vi "GFITS_NetServer2.vi"(7 "ID":string, 8 "error in (no error)":errorcluster, 9 "notifier In":refnum<notifier>, 10 "messages from sock":refnum<queue>, 11 "listener ID":refnum<k5>) -> (0 "error out":errorcluster)   [LabVIEW 2016]
uses:
  DHS_TCPSERVER_MsgStruct.ctl
panel:
  in  "ResponseStruct":T1
  out "sock ID":refnum<k5>
  out "stop":bool
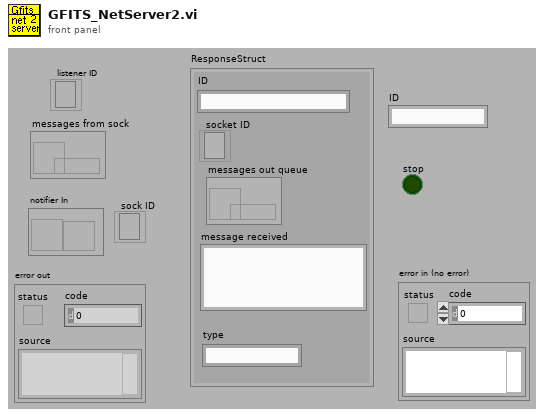
[diagram p1: front panel]
types:
  T1 = typedef "DHS_TCPSERVER_MsgStruct.ctl" = cluster{"ID":string, "socket ID":refnum<k5>, "messages out queue":refnum<queue>, "message received":string, "type":string}
  T2 = enum16{"Standard", "Buffered", "CRLF", "Immediate"}
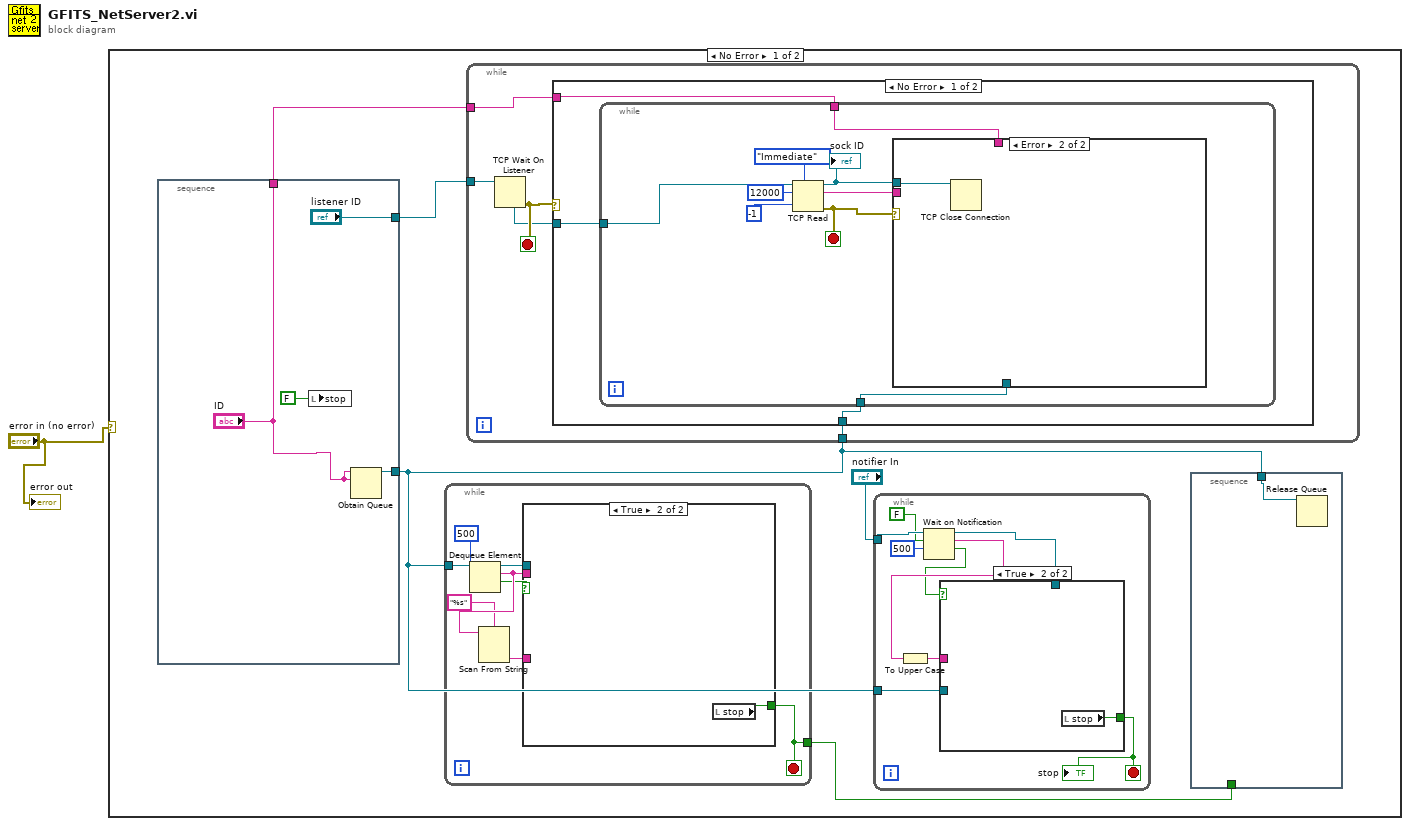
[diagram p0: block diagram]
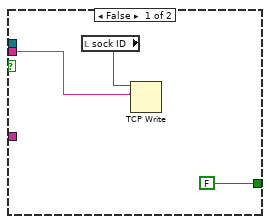
[diagram p2: hidden frame]
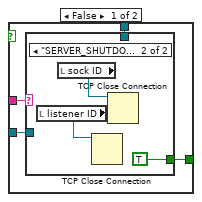
[diagram p3: hidden frame]
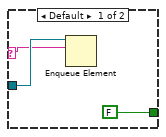
[diagram p4: hidden frame]
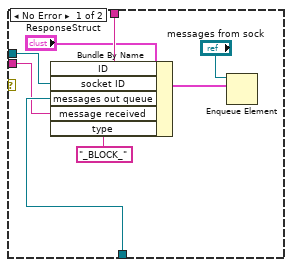
[diagram p5: hidden frame]
diagram:
  n1 = case shown="No Error" "error in (no error)" {
    frame No Error {
      n2 = stacked-sequence {
        tunnel: [w11] -> w2
        tunnel: ["listener ID"] -> w5
        tunnel: ["ID"] -> w4
        frame #0 {
          n3 = local write "stop"(FALSE ("stop")) -> ()
          n4 = Obtain Queue(name (unnamed)="ID", element data type="ID") -> (queue out=w11:refnum<queue>)  [unwired: 3 in, 2 out]
        }
      }
      n5 = while {
        tunnel: w2 -> [w19]
        tunnel: [w12] -> w3
        stop <- w12 stop-if-true
        n6 = Dequeue Element(queue=w19, timeout in ms (-1)=500) -> (queue out=w15:refnum<queue>, element=w18:string, timed out?=w14:bool)  [unwired: 1 in, 1 out]
        n7 = Scan From String(format string="%s", input string=w18) -> (output 1=w16:string)  [unwired: 2 in, 4 out]
        n8 = case shown="True" w14 {
          tunnel: w18 -> [w22 _]
          tunnel: w16 -> [_ _]
          tunnel: [FALSE w23] -> w12
          tunnel: w15 -> [_ _]
          frame False {
            n9 = local read "sock ID"() -> (w20:refnum<k5>)
            n10 = TCP Write(connection ID=w20, data in=w22) -> ()  [unwired: 1 in, 4 out]
          }
          frame True {
            n11 = local read "stop"() -> (w23:bool)
          }
        }
      }
      n12 = while {
        tunnel: w5 -> [w48]
        tunnel: w2 -> [w45]
        tunnel: w4 -> [w44]
        stop <- w47 stop-if-true
        n13 = TCP Wait On Listener(11:w48) -> (0:w47:errorcluster, 4:w46:refnum<k5>)  [unwired: 1 in, 5 out]
        n14 = case shown="No Error" w47 {
          tunnel: w46 -> [w51 _]
          tunnel: w45 -> [w50 _]
          tunnel: w44 -> [w49 _]
          frame No Error {
            n15 = while {
              tunnel: w51 -> [w54]
              tunnel: w50 -> [w55]
              tunnel: w49 -> [w56]
              stop <- w59 stop-if-true
              n16 = TCP Read(connection ID=w54, bytes to read=12000, 7:T2."Immediate" ("mode (standard)"), 9:-1 ("timeout ms (25000)")) -> (connection ID out=w57:refnum<k5>, data out=w58:string, error out=w59:errorcluster)  [unwired: 1 in]
              "sock ID" <- w57
              n17 = case shown="Error" w59 {
                tunnel: w58 -> [w64 _]
                tunnel: w55 -> [w66 _]
                tunnel: w57 -> [w68 w69]
                tunnel: w56 -> [w67 _]
                frame No Error {
                  n18 = Bundle By Name(cluster="ResponseStruct", "ID"=w67, "socket ID"=w68, "messages out queue"=w66, "message received"=w64, "type"="_BLOCK_") -> (w61:T1)
                  n19 = Enqueue Element(queue="messages from sock", element=w61) -> ()  [unwired: 1 in, 4 out]
                }
                frame Error {
                  n20 = TCP Close Connection(connection ID=w69) -> ()  [unwired: 1 in, 3 out]
                }
              }
            }
          }
          frame Error {
          }
        }
      }
      n21 = while {
        tunnel: "notifier In" -> [w32]
        tunnel: w2 -> [w27]
        stop <- w24 stop-if-true
        n22 = Wait on Notification(notifier=w32, ignore previous (F)=FALSE, timeout in ms (-1)=500) -> (notifier out=w30:refnum<notifier>, notification=w29:string, timed out?=w25:bool)  [unwired: 1 in, 1 out]
        n23 = To Upper Case(1:w29) -> (0:w28:string)
        n24 = case shown="True" w25 {
          tunnel: w30 -> [w36 _]
          tunnel: w28 -> [w35 _]
          tunnel: [w34 w43] -> w24
          tunnel: w27 -> [w33 _]
          frame False {
            n25 = case shown="\"SERVER_SHUTDOWN\"" w35 {
              selector: w35 -> [w37 _]
              tunnel: w36 -> [_ _]
              tunnel: [FALSE TRUE] -> w34
              tunnel: w33 -> [w38 _]
              frame Default {
                n26 = Enqueue Element(queue=w38, element=w37) -> ()  [unwired: 1 in, 4 out]
              }
              frame "SERVER_SHUTDOWN" {
                n27 = local read "listener ID"() -> (w40:refnum<k5>)
                n28 = local read "sock ID"() -> (w41:refnum<k5>)
                n29 = TCP Close Connection(connection ID=w40) -> ()  [unwired: 1 in, 3 out]
                n30 = TCP Close Connection(connection ID=w41) -> ()  [unwired: 1 in, 3 out]
              }
            }
          }
          frame True {
            n31 = local read "stop"() -> (w43:bool)
          }
        }
        "stop" <- w24
      }
      n32 = stacked-sequence {
        tunnel: w3 -> [_]
        tunnel: w2 -> [w7]
        frame #0 {
          n33 = Release Queue(queue=w7) -> ()  [unwired: 1 in, 4 out]
        }
      }
    }
    frame Error {
    }
  }
  "error out" <- "error in (no error)"
